vi "Resize Combobox.vi"(8 "error in (no error)":errorcluster, 9 "Cmb Box":refnum<vi>, 10 "Bounds":T1, 11 "Path Selector in":refnum<class "MGI Path Selector.lvclass">) -> (0 "error out":errorcluster, 2 "Changed?":bool, 3 "Path Selector out":refnum<class "MGI Path Selector.lvclass">)   [LabVIEW 2016, in "MGI Path Selector.lvclass"]
doc: "Resize the specified Combobox to match the specified Bounds.\n\nAuthored by Shawn Walpole\nsupport@mooregoodideas.com\nwww.mooregoodideas.com\n\nCopyright (c) 2013, Moore Good Ideas, Inc.\n\nAll rights reserved.\n\nRedistribution and use in source and binary forms, with or without modification, are permitted provided that the following conditions are met:\n\n * Redistributions of source code must retain the above copyright notice, this list of conditions and the following disclaimer.\n * Redistributions in binary form must reproduce the above copyright notice, this list of conditions and the following disclaimer in the documentation and/or other materials provided with the distribution.\n * Neither the name of Moore Good Ideas, Inc. nor the names of its contributors may be used to endorse or promote products derived from this software without specific prior written permission.\n\nTHIS SOFTWARE IS PROVIDED BY THE COPYRIGHT HOLDERS AND CONTRIBUTORS \"AS IS\" AND ANY EXPRESS OR IMPLIED WARRANTIES, INCLUDING, BUT NOT LIMITED TO, THE IMPLIED WARRANTIES OF MERCHANTABILITY AND FITNESS FOR A PARTICULAR PURPOSE ARE DISCLAIMED. IN NO EVENT SHALL THE COPYRIGHT OWNER OR CONTRIBUTORS BE LIABLE FOR ANY DIRECT, INDIRECT, INCIDENTAL, SPECIAL, EXEMPLARY, OR CONSEQUENTIAL DAMAGES (INCLUDING, BUT NOT LIMITED TO, PROCUREMENT OF SUBSTITUTE GOODS OR SERVICES; LOSS OF USE, DATA, OR PROFITS; OR BUSINESS INTERRUPTION) HOWEVER CAUSED AND ON ANY THEORY OF LIABILITY, WHETHER IN CONTRACT, STRICT LIABILITY, OR TORT (INCLUDING NEGLIGENCE OR OTHERWISE) ARISING IN ANY WAY OUT OF THE USE OF THIS SOFTWARE, EVEN IF ADVISED OF THE POSSIBILITY OF SUCH DAMAGE."
uses:
  <userlib>/_MGI/User Interface/Path Selector XControl/Class Hierarchy/MGI Path Selector.lvclass
  <vilib>/Utility/miscctls.llb/LVRectTypeDef.ctl
  <userlib>/_MGI/User Interface/Path Selector XControl/Control Style Enum.ctl
  <userlib>/_MGI/User Interface/Path Selector XControl/MGI Path Selector.xctl
panel:
  in  "Size Adjust":cluster{"x":i16, "y":i16}={"x"=-10, "y"=-10}
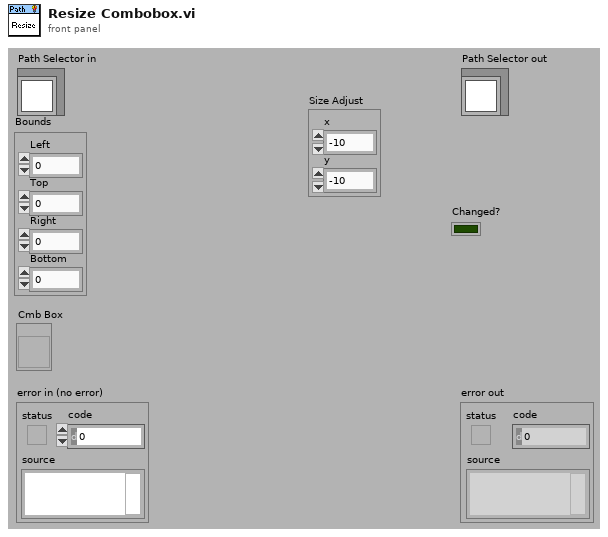
[diagram p1: front panel]
types:
  T1 = typedef "LVRectTypeDef.ctl" = cluster{"Left":i16, "Top":i16, "Right":i16, "Bottom":i16}
  T2 = typedef "MGI Path Selector.xctl/Control Style Enum.ctl" = enum16{"System", "Modern", "Classic", "Silver"}
  T3 = typedef "LVBoundsTypeDef.ctl" = cluster{"Width":u32, "Height":u32}
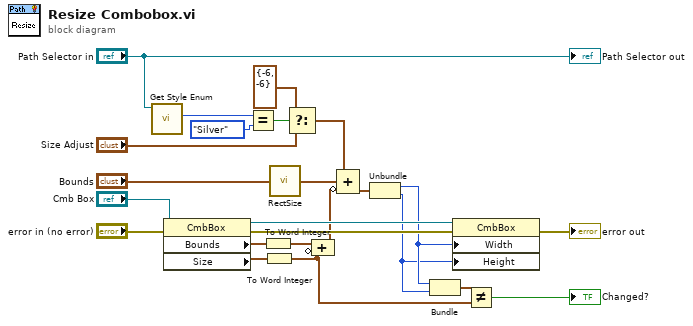
[diagram p0: block diagram]
diagram:
  n1 = call-dynamic "Get Style Enum.vi"("Path Selector in"="Path Selector in") -> ("Control Style"=w6:T2)  [unwired: 10 in]
  n2 = property on="Property Node" class="CmbBox"(reference="Cmb Box", error in="error in (no error)") -> (reference out=w19:refnum<vi>, error out=w18:errorcluster, "Bounds"=w23:T3, "Size"=w22:T3)
  n3 = Equal?(x=w6, y=Control_Style_Enum."Silver") -> (x = y?=w4:bool)
  n4 = To Word Integer(number=w23) -> (16bit integer=w24:cluster{"Width":i16, "Height":i16})
  n5 = To Word Integer(number=w22) -> (16bit integer=w8:cluster{"Width":i16, "Height":i16})
  n6 = call <vilib>:"RectSize.vi"("rect"="Bounds") -> ("point"=w20:cluster{"x":i16, "y":i16})
  n7 = Select(t=cluster{"x":i16, "y":i16} {"x"=-6, "y"=-6}, s=w4, f="Size Adjust") -> (s? t:f=w2:cluster{"x":i16, "y":i16})
  n8 = Compound Arithmetic op=ADD(w24, invert w8) -> (w11:cluster{"Width":i16, "Height":i16})
  n9 = Compound Arithmetic op=ADD(w2, w20, invert w11) -> (w21:cluster{i16, i16})
  n10 = Unbundle(w21) -> (w13:i16, w12:i16)
  n11 = Bundle(w13, w12) -> (w10:cluster{i16, i16})  [unwired: 1 in]
  n12 = property class="CmbBox"(reference=w19, error in=w18, "Width"=w13, "Height"=w12) -> (error out=→"error out":errorcluster)  [unwired: 1 out]
  n13 = Not Equal?(x=w10, y=w8) -> (x != y?=→"Changed?":bool)
  "Path Selector out" <- "Path Selector in"
